vi "Read Tournament Stat.vi"(10 "Stat Name":string, 11 "Tournament Data In in":string) -> (2 "Remaining String Out":string, 3 "Stat Value":i32)   [LabVIEW 2020]
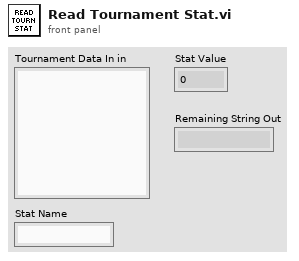
[diagram p1: front panel]
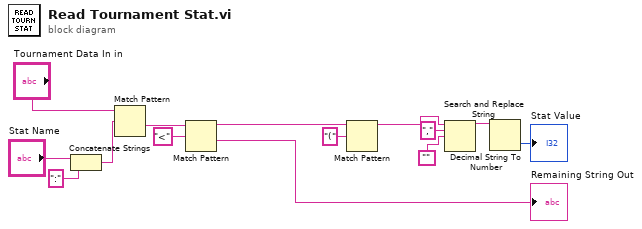
[diagram p0: block diagram]
diagram:
  n1 = Concatenate Strings("Stat Name", ":" ("string")) -> (w5:string)
  n2 = Match Pattern(string="Tournament Data In in", regular expression=w5) -> (after substring=w9:string)  [unwired: 1 in, 3 out]
  n3 = Match Pattern(string=w9, regular expression="<" ("y")) -> (before substring=w3:string, after substring=→"Remaining String Out":string)  [unwired: 1 in, 2 out]
  n4 = Match Pattern(string=w3, regular expression="(") -> (before substring=w1:string)  [unwired: 1 in, 3 out]
  n5 = Search and Replace String(input string=w1, search string=",", replace string="") -> (result string=w14:string)  [unwired: 5 in, 3 out]
  n6 = Decimal String To Number(string=w14) -> (number=→"Stat Value":i32)  [unwired: 2 in, 1 out]
